vi "Ack_Nack Bit.vi"(8 "error in (no error)":errorcluster, 11 "Low Speed in":refnum<class "Low Speed.lvclass">) -> (0 "error out":errorcluster, 3 "Low Speed out":refnum<class "Low Speed.lvclass">)   [LabVIEW 2020, in "Low Speed.lvclass"]
uses:
  Low Speed.lvclass
  C:/Users/kaiser.asan/OneDrive - SolitonTechnologies/LabVIEW/29.SDLC - I2C Driver/I2C Module/I2C Controller Module/Class/Transmission Mode/Parent/TX Speed.lvclass
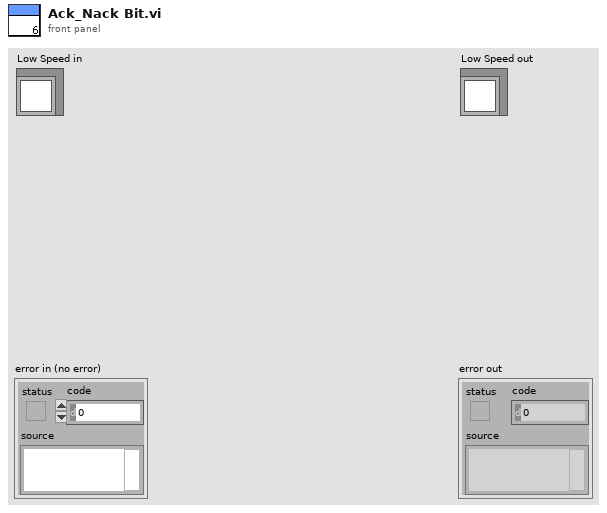
[diagram p1: front panel]
types:
  T1 = typedef "I2C Controller Lib.lvlib/Timing Parameters Cluster.ctl" = cluster{"f_SCL(KHz)":u32, "t_HIGH (ns)":u32, "t_LOW (ns)":u32, "t_SU;STA (ns)":u32, "t_HD;STA (ns)":u32, "t_SU;DAT (ns)":u32, "t_HD;DAT (ns)":u32, "t_SU;STO (ns)":u32, "t_BUF (ns)":u32}
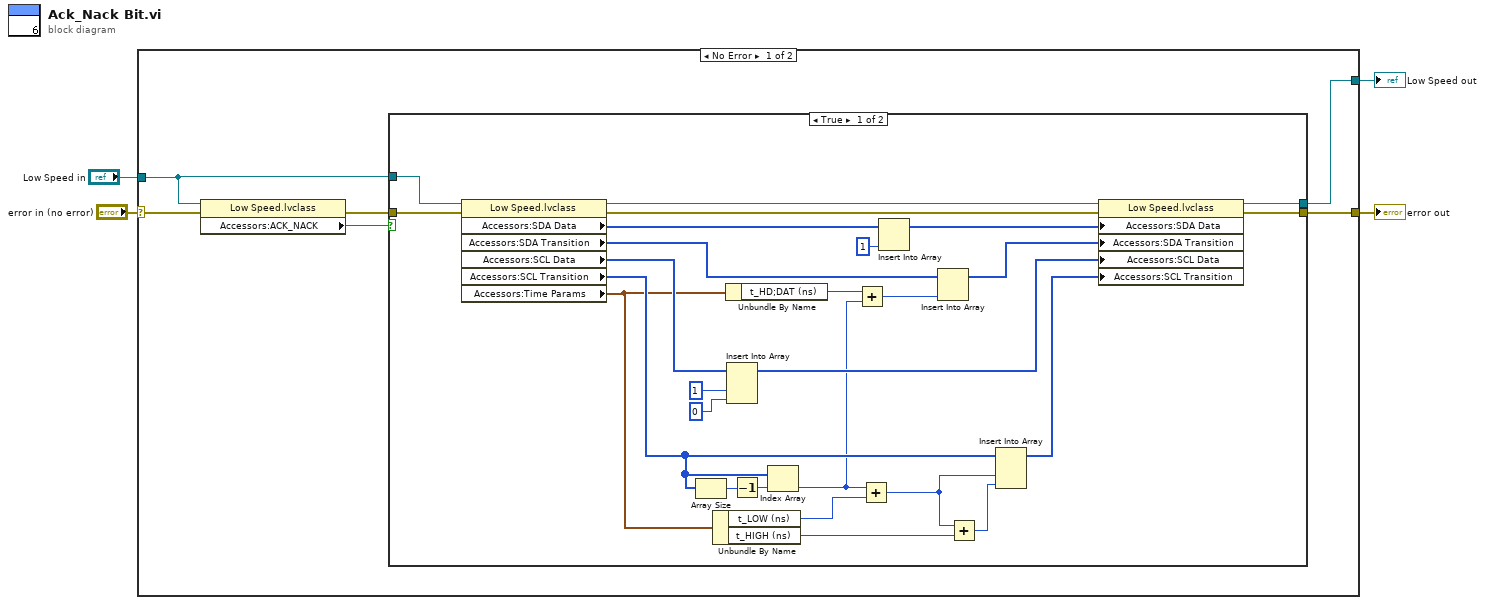
[diagram p0: block diagram]
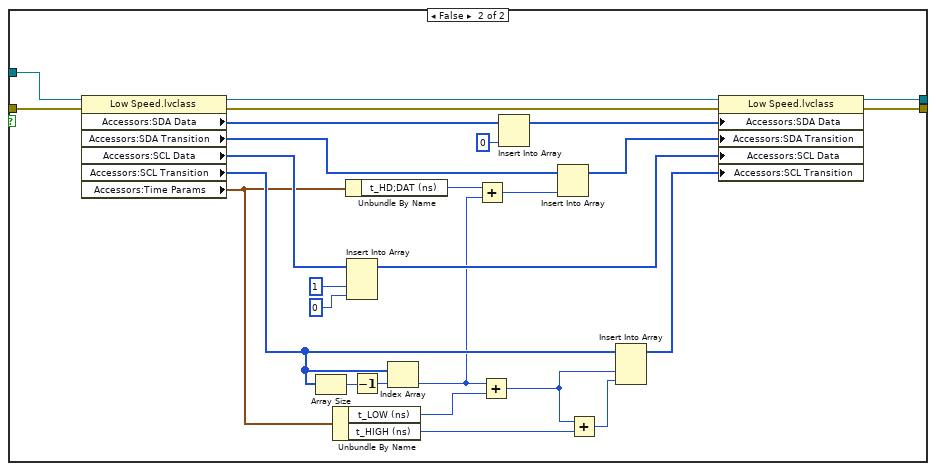
[diagram p2: hidden frame]
diagram:
  n1 = case shown="No Error" "error in (no error)" {
    selector: "error in (no error)" -> [w10 w66]
    tunnel: [w8 w66] -> w4
    tunnel: [w7 w65] -> w3
    tunnel: "Low Speed in" -> [w9 w65]
    frame No Error {
      n2 = property class="Low Speed.lvclass"(reference=w9, error in=w10) -> (error out=w5:errorcluster, "Accessors:ACK_NACK"=w6:bool)  [unwired: 1 out]
      n3 = case shown="True" w6 {
        tunnel: w5 -> [w14 w41]
        tunnel: w9 -> [w12 w39]
        tunnel: [w13 w40] -> w8
        tunnel: [w11 w38] -> w7
        frame True {
          n4 = property class="Low Speed.lvclass"(reference=w12, error in=w14) -> (reference out=w34:refnum<class "Low Speed.lvclass">, error out=w37:errorcluster, "Accessors:SDA Data"=w23:u8[], "Accessors:SDA Transition"=w18:u32[], "Accessors:SCL Data"=w33:u8[], "Accessors:SCL Transition"=w25:u32[], "Accessors:Time Params"=w19:T1)
          n5 = Array Size(array=w25) -> (size(s)=w31:i32)
          n6 = Unbundle By Name(w19) -> ("t_LOW (ns)"=w29:u32, "t_HIGH (ns)"=w28:u32)
          n7 = Unbundle By Name(w19) -> ("t_HD;DAT (ns)"=w16:u32)
          n8 = Insert Into Array(array=w33, new element #1=u8 1 ("new element/subarray"), new element #2=u8 0 ("new element/subarray")) -> (w32:u8[])  [unwired: 1 in]
          n9 = Decrement(x=w31) -> (x-1=w30:i32)
          n10 = Index Array(array=w25, index=w30) -> (element=w15:u32)
          n11 = Add(x=w16, y=w15) -> (x+y=w20:u32)
          n12 = Add(x=w15, y=w29) -> (x+y=w26:u32)
          n13 = Insert Into Array(array=w23, new element=u8 1 ("new element/subarray")) -> (w22:u8[])  [unwired: 1 in]
          n14 = Insert Into Array(array=w18, new element=w20) -> (w17:u32[])  [unwired: 1 in]
          n15 = Add(x=w26, y=w28) -> (x+y=w27:u32)
          n16 = Insert Into Array(array=w25, new element #1=w26, new element #2=w27) -> (w24:u32[])  [unwired: 1 in]
          n17 = property class="Low Speed.lvclass"(reference=w34, error in=w37, "Accessors:SDA Data"=w22, "Accessors:SDA Transition"=w17, "Accessors:SCL Data"=w32, "Accessors:SCL Transition"=w24) -> (reference out=w11:refnum<class "Low Speed.lvclass">, error out=w13:errorcluster)
        }
        frame False {
          n18 = property class="Low Speed.lvclass"(reference=w39, error in=w41) -> (reference out=w61:refnum<class "Low Speed.lvclass">, error out=w64:errorcluster, "Accessors:SDA Data"=w50:u8[], "Accessors:SDA Transition"=w45:u32[], "Accessors:SCL Data"=w60:u8[], "Accessors:SCL Transition"=w52:u32[], "Accessors:Time Params"=w46:T1)
          n19 = Array Size(array=w52) -> (size(s)=w58:i32)
          n20 = Unbundle By Name(w46) -> ("t_LOW (ns)"=w56:u32, "t_HIGH (ns)"=w55:u32)
          n21 = Unbundle By Name(w46) -> ("t_HD;DAT (ns)"=w43:u32)
          n22 = Insert Into Array(array=w60, new element #1=u8 1 ("new element/subarray"), new element #2=u8 0 ("new element/subarray")) -> (w59:u8[])  [unwired: 1 in]
          n23 = Decrement(x=w58) -> (x-1=w57:i32)
          n24 = Index Array(array=w52, index=w57) -> (element=w42:u32)
          n25 = Add(x=w43, y=w42) -> (x+y=w47:u32)
          n26 = Add(x=w42, y=w56) -> (x+y=w53:u32)
          n27 = Insert Into Array(array=w50, new element=u8 0 ("new element/subarray")) -> (w49:u8[])  [unwired: 1 in]
          n28 = Insert Into Array(array=w45, new element=w47) -> (w44:u32[])  [unwired: 1 in]
          n29 = Add(x=w53, y=w55) -> (x+y=w54:u32)
          n30 = Insert Into Array(array=w52, new element #1=w53, new element #2=w54) -> (w51:u32[])  [unwired: 1 in]
          n31 = property class="Low Speed.lvclass"(reference=w61, error in=w64, "Accessors:SDA Data"=w49, "Accessors:SDA Transition"=w44, "Accessors:SCL Data"=w59, "Accessors:SCL Transition"=w51) -> (reference out=w38:refnum<class "Low Speed.lvclass">, error out=w40:errorcluster)
        }
      }
    }
    frame Error {
    }
  }
  "error out" <- w4
  "Low Speed out" <- w3
